vi "WriteFile.vi"(0 "refnum":T1, 1 "Frequency":T9={"FrequencyStart"=5000.0, "FrequencyStop"=10000.0, "FrequencyOffset"=0.0}, 2 "Level":T6={"InputImpedance"=50.0, "AttenuationAuto"=FALSE, "ReferenceLevel"=0.0, "Attenuation"=0.0, "ReferenceLevelOffset"=0.0, "amplitude units (dBm)"=1} {"amplitude units (dBm)" items=["dBm"=1, "dBmV"=2, "dBuV"=3, "dBuA"=1001, "Volt"=4, "Watt"=5, "Amper"=1002]}, 3 "SweepCoupling":T8={"ResolutionBandwidth"=3000000.0, "ResolutionBandwidthAuto"=TRUE, "SweepTime"=0.004, "VideoBandwidth"=300000.0, "VideoBandwidthAuto"=TRUE, "SweepTimeAuto"=TRUE}, 4 "Trace":T7=[{"TraceName"="TRACE1", "TraceSize"=200, "TraceType"=1}] {"TraceType" items=["Clear Write"=1, "Maximum Hold"=2, "Minimum Hold"=3, "View"=4, "Store"=5, "Video Average"=6]}, 5 "error in (no error)":errorcluster, 6 "Acquisition":T10={"Handle"="who", "Connected"=FALSE, "Enabled"=TRUE, "SweepModeContinuous"=TRUE, "NumberOfSweeps"=1, "DetectorTypeAuto"=TRUE, "DetectorType"=2, "VerticalScale"=1, "MaximumTime(seconds)"=1.0} {"VerticalScale" items=["Linear", "Logarithmic"]; "DetectorType" items=["AutoPeak", "Average", "MaximumPeak", "MinimumPeak", "Sample", "RMS"]}, 7 "Marker":T2={"MarkerEnabled"=TRUE, "MarkerThreshold"=0.0, "PeakExcursion"=0.0, "SignalTrackEnabled"=FALSE, "MarkerPosition"=7500.0, "Instrument Setting (Frequency Center)"=3, "Marker search (Minimum)"=2, "ActiveMarker"="MARKER1", "MarkerFrequencyCounter"=FALSE, "FrequencyCounterResolution"=0.0} {"Marker search (Minimum)" items=["Highest"=1, "Next Peak"=3, "Next Peak Left"=4, "Next Peak Right"=5, "Minimum"=2]; "Instrument Setting (Frequency Center)" items=["Frequency Start"=3, "Frequency Stop"=4, "Frequency Center"=1, "Frequency Span"=2, "Reference Level"=5]}, 8 "section":string, 9 "Trigger":T5={"TriggerLevel"=0.0, "TriggerSlope"=1, "Trigger Source"=2} {"Trigger Source" items=["External"=1, "Immediate"=2, "AC Line"=4, "Video"=5, "TV"=1001, "RF Burst"=1002]; "TriggerSlope" items=["Positive"=1, "Negative"=2]}, 11 "RF Burst":T4={"Frequency Selectivity (OFF)"=FALSE, "Trigger Level Type (Absolute)"=1, "Narrow Pulse Discriminator (OFF)"=FALSE} {"Trigger Level Type (Absolute)" items=["Absolute"=1, "Relative"=2]}, 13 "TV":T3={"Monitor Enabled (OFF)"=FALSE, "SynchronizeSweep"=FALSE, "SynchronizationLineNumber"=0, "TV Field (Any Field)"=3, "TV Signal Format (NTSC-M)"=1, "Trigger Source (Spectrum Analyzer)"=2} {"Trigger Source (Spectrum Analyzer)" items=["External"=1, "Spectrum Analyzer"=2]; "TV Signal Format (NTSC-M)" items=["NTSC-M"=1, "NTSC-Japan"=2, "PAL-M"=3, "PAL-B,D,G,H,I"=4, "PAL-N"=5, "PAL-N Combin"=6, "SECAM-L"=7]; "TV Field (Any Field)" items=["Field 1"=1, "Field 2"=2, "Any Field"=3]}) -> (19 "error out":errorcluster)   [LabVIEW 2018, in "SpecAnPlugins.lvlib" / "Keysight44xx.lvclass"]
uses:
  Keysight44xx.lvclass
  SpecAnBaseClass/Typedefs/Acquisition.ctl
  SpecAnBaseClass/Typedefs/Frequency.ctl
  SpecAnBaseClass/Typedefs/SweepCoupling.ctl
  SpecAnBaseClass/Typedefs/Trace.ctl
  SpecAnBaseClass/Typedefs/Level.ctl
  SpecAnBaseClass/Typedefs/Trigger.ctl
  TypeDefs/RFBurst.ctl
  TypeDefs/TV.ctl
  SpecAnBaseClass/Typedefs/Markers.ctl
  <vilib>/Utility/config.llb/Config Data RefNum.ctl
  <vilib>/Utility/config.llb/NI_LVConfig.lvlib
  SpecAnBaseClass/SpecAnBase.lvclass
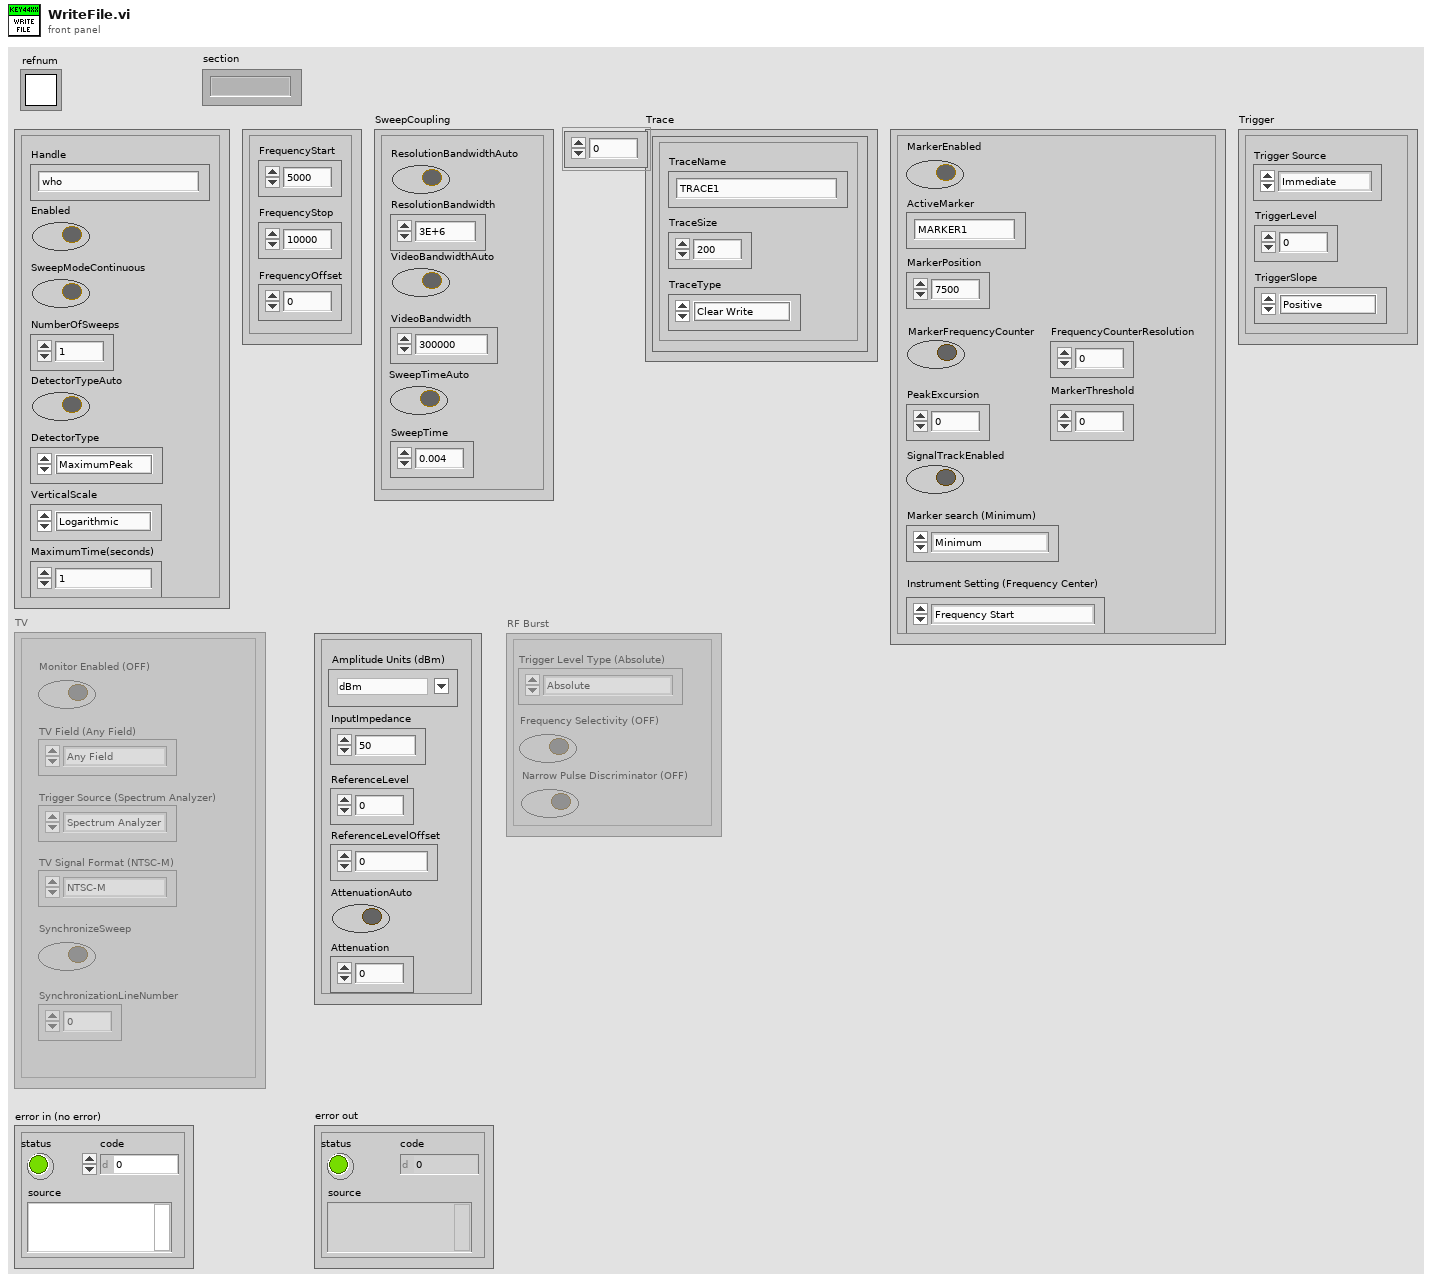
[diagram p1: front panel]
types:
  T1 = typedef "NI_LVConfig.lvlib/Config Data RefNum.ctl" = refnum<k1>
  T2 = typedef "SpecAnPlugins.lvlib/SpecAnBase.lvclass/Markers.ctl" = cluster{"MarkerEnabled":bool, "MarkerThreshold":dbl, "PeakExcursion":dbl, "SignalTrackEnabled":bool, "MarkerPosition":dbl, "Instrument Setting (Frequency Center)":i32, "Marker search (Minimum)":i32, "ActiveMarker":string, "MarkerFrequencyCounter":bool, "FrequencyCounterResolution":dbl}
  T3 = typedef "SpecAnPlugins.lvlib/Keysight44xx.lvclass/TV.ctl" = cluster{"Monitor Enabled (OFF)":bool, "SynchronizeSweep":bool, "SynchronizationLineNumber":i32, "TV Field (Any Field)":i32, "TV Signal Format (NTSC-M)":i32, "Trigger Source (Spectrum Analyzer)":i32}
  T4 = typedef "SpecAnPlugins.lvlib/Keysight44xx.lvclass/RFBurst.ctl" = cluster{"Frequency Selectivity (OFF)":bool, "Trigger Level Type (Absolute)":i32, "Narrow Pulse Discriminator (OFF)":bool}
  T5 = typedef "SpecAnPlugins.lvlib/SpecAnBase.lvclass/Trigger.ctl" = cluster{"TriggerLevel":dbl, "TriggerSlope":i32, "Trigger Source":i32}
  T6 = typedef "SpecAnPlugins.lvlib/SpecAnBase.lvclass/Level.ctl" = cluster{"InputImpedance":dbl, "AttenuationAuto":bool, "ReferenceLevel":dbl, "Attenuation":dbl, "ReferenceLevelOffset":dbl, "amplitude units (dBm)":i32}
  T7 = typedef "SpecAnPlugins.lvlib/SpecAnBase.lvclass/Trace.ctl" = cluster{"TraceName":string, "TraceSize":i32, "TraceType":i32}[]
  T8 = typedef "SpecAnPlugins.lvlib/SpecAnBase.lvclass/SweepCoupling.ctl" = cluster{"ResolutionBandwidth":dbl, "ResolutionBandwidthAuto":bool, "SweepTime":dbl, "VideoBandwidth":dbl, "VideoBandwidthAuto":bool, "SweepTimeAuto":bool}
  T9 = typedef "SpecAnPlugins.lvlib/SpecAnBase.lvclass/Frequency.ctl" = cluster{"FrequencyStart":dbl, "FrequencyStop":dbl, "FrequencyOffset":dbl}
  T10 = typedef "SpecAnPlugins.lvlib/SpecAnBase.lvclass/Acquisition.ctl" = cluster{"Handle":string, "Connected":bool, "Enabled":bool, "SweepModeContinuous":bool, "NumberOfSweeps":i32, "DetectorTypeAuto":bool, "DetectorType":i32, "VerticalScale":i32, "MaximumTime(seconds)":dbl}
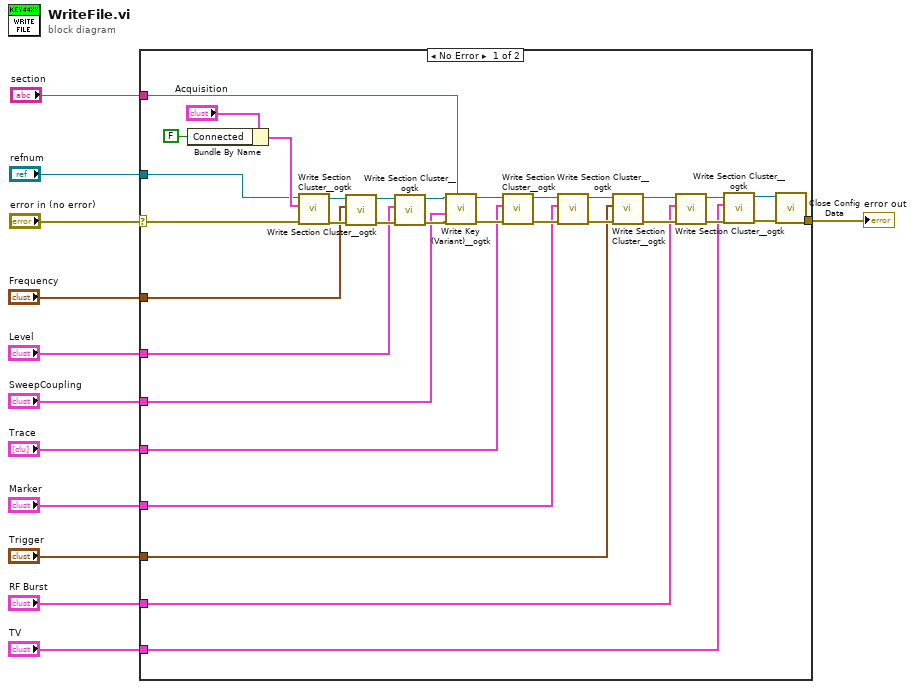
[diagram p0: block diagram]
diagram:
  n1 = case shown="No Error" "error in (no error)" {
    selector: "error in (no error)" -> [w30 w46]
    tunnel: [w31 w46] -> w12
    tunnel: "Frequency" -> [w29 _]
    tunnel: "Level" -> [w28 _]
    tunnel: "SweepCoupling" -> [w27 _]
    tunnel: "Trace" -> [w26 _]
    tunnel: "Marker" -> [w25 _]
    tunnel: "Trigger" -> [w24 _]
    tunnel: "RF Burst" -> [w23 _]
    tunnel: "TV" -> [w18 _]
    tunnel: "refnum" -> [w14 _]
    tunnel: "section" -> [w13 _]
    frame No Error {
      n2 = Bundle By Name(cluster="Acquisition", "Connected"=FALSE) -> (w15:T10)
      n3 = call <userlib>:"Write Section Cluster__ogtk.vi"("error in (no error)"=w30, "Section Formatted Cluster"=w15, "refnum"=w14) -> ("error out"=w45:errorcluster, "dup refnum"=w44:T1)  [unwired: 7 in]
      n4 = call <userlib>:"Write Section Cluster__ogtk.vi"("error in (no error)"=w45, "Section Formatted Cluster"=w29, "refnum"=w44) -> ("error out"=w43:errorcluster, "dup refnum"=w42:T1)  [unwired: 7 in]
      n5 = call <userlib>:"Write Section Cluster__ogtk.vi"("error in (no error)"=w43, "Section Formatted Cluster"=w28, "refnum"=w42) -> ("error out"=w41:errorcluster, "dup refnum"=w40:T1)  [unwired: 7 in]
      n6 = call <userlib>:"Write Key (Variant)__ogtk.vi"("section"=w13, "error in (no error)"=w41, "key-value"=w27, "refnum"=w40) -> ("error out"=w39:errorcluster, "refnum out"=w38:T1)  [unwired: 6 in]
      n7 = call <userlib>:"Write Section Cluster__ogtk.vi"("error in (no error)"=w39, "Section Formatted Cluster"=w26, "refnum"=w38) -> ("error out"=w35:errorcluster, "dup refnum"=w34:T1)  [unwired: 7 in]
      n8 = call <userlib>:"Write Section Cluster__ogtk.vi"("error in (no error)"=w35, "Section Formatted Cluster"=w25, "refnum"=w34) -> ("error out"=w33:errorcluster, "dup refnum"=w32:T1)  [unwired: 7 in]
      n9 = call <userlib>:"Write Section Cluster__ogtk.vi"("error in (no error)"=w33, "Section Formatted Cluster"=w24, "refnum"=w32) -> ("error out"=w37:errorcluster, "dup refnum"=w36:T1)  [unwired: 7 in]
      n10 = call <userlib>:"Write Section Cluster__ogtk.vi"("error in (no error)"=w37, "Section Formatted Cluster"=w23, "refnum"=w36) -> ("error out"=w22:errorcluster, "dup refnum"=w21:T1)  [unwired: 7 in]
      n11 = call <userlib>:"Write Section Cluster__ogtk.vi"("error in (no error)"=w22, "Section Formatted Cluster"=w18, "refnum"=w21) -> ("error out"=w20:errorcluster, "dup refnum"=w19:T1)  [unwired: 7 in]
      n12 = call <vilib>:"Close Config Data.vi"("error in (no error)"=w20, "refnum"=w19) -> ("error out"=w31:errorcluster)  [unwired: 8 in, 1 out]
    }
    frame Error {
    }
  }
  "error out" <- w12
